vi "Read Dashboard Buttons.vi"(7 "timeout in ms (-1)":i32=-1, 8 "error in":errorcluster, 11 "CAN Session In":T1=refnum) -> (0 "error out":errorcluster, 1 "Tractive system activation":bool, 2 "Ready to drive":bool, 3 "CAN Session Out":T1)   [LabVIEW 2016]
uses:
  Program Files (x86)/National Instruments/LabVIEW 2016/examples/robotics/EPOS2 CANOpen Driver/Low Level VIs/Typedefs/CAN Refnum.ctl
  Program Files (x86)/National Instruments/LabVIEW 2016/examples/robotics/EPOS2 CANOpen Driver/Low Level VIs/Typedefs/CAN Session Pointer.ctl
  Program Files (x86)/National Instruments/LabVIEW 2016/examples/robotics/EPOS2 CANOpen Driver/Low Level VIs/Typedefs/CAN Communication References.ctl
  Program Files (x86)/National Instruments/LabVIEW 2016/examples/robotics/EPOS2 CANOpen Driver/Low Level VIs/Typedefs/kill process notifier array.ctl
  Program Files (x86)/National Instruments/LabVIEW 2016/examples/robotics/EPOS2 CANOpen Driver/Low Level VIs/Typedefs/Write Queue.ctl
  Program Files (x86)/National Instruments/LabVIEW 2016/examples/robotics/EPOS2 CANOpen Driver/Low Level VIs/Typedefs/FPGA CAN Frame Cluster.ctl
  RT/Read single CAN.vi
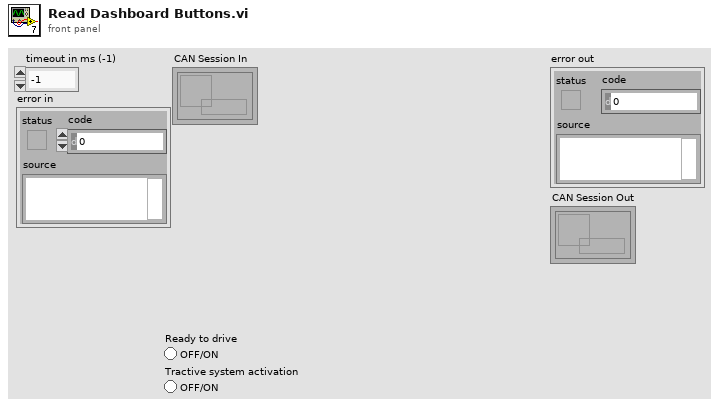
[diagram p1: front panel]
types:
  T1 = typedef "CAN Refnum.ctl" = refnum<k1>
  T2 = typedef "FPGA CAN Frame Cluster.ctl" = cluster{"Timestamp":u64, "Identifier":u32, "Type":u8, "InfoA":u8, "InfoB":u8, "DataLength":u8, "Data":u8[]}
  T3 = cluster{"Boolean array[0]":bool, "Boolean array[1]":bool, "Boolean array[2]":bool, "Boolean array[3]":bool, "Boolean array[4]":bool, "Boolean array[5]":bool, "Boolean array[6]":bool, "Boolean array[7]":bool, "Boolean array[8]":bool}
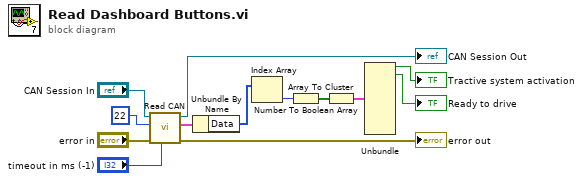
[diagram p0: block diagram]
diagram:
  n1 = call-poly "Read CAN.vi"("timeout in ms (-1)"="timeout in ms (-1)", "error in"="error in", "ID"=22, "CAN Session In"="CAN Session In") -> ("error out"=→"error out":errorcluster, "CAN Frame Out"=w7:T2, "CAN Session Out"=→"CAN Session Out":T1)  [unwired: 5 in]
  n2 = Unbundle By Name(w7) -> ("Data"=w6:u8[])
  n3 = Index Array(array=w6) -> (element=w11:u8)  [unwired: 1 in]
  n4 = Number To Boolean Array(number=w11) -> (Boolean array=w10:bool[])
  n5 = Array To Cluster(array=w10) -> (cluster=w12:T3)
  n6 = Unbundle(w12) -> ("Boolean array[0]"=→"Tractive system activation":bool, "Boolean array[1]"=→"Ready to drive":bool)  [unwired: 7 out]
